vi "Access Integer.vi"(7 "Get/Set":enum16{"Get", "Set"}(ring), 8 "error in (no error)":errorcluster, 9 "Value in":i32, 10 "Key":string, 11 "FlexWorktable in":refnum<class "FlexWorktable.lvclass">) -> (0 "error out":errorcluster, 1 "Value out":i32, 3 "FlexWorktable out":refnum<class "FlexWorktable.lvclass">)   [LabVIEW 2017, in "FlexWorktable.lvclass"]
uses:
  FlexWorktable.lvclass
  FlexWorktable.lvclass/FlexWorktable.ctl
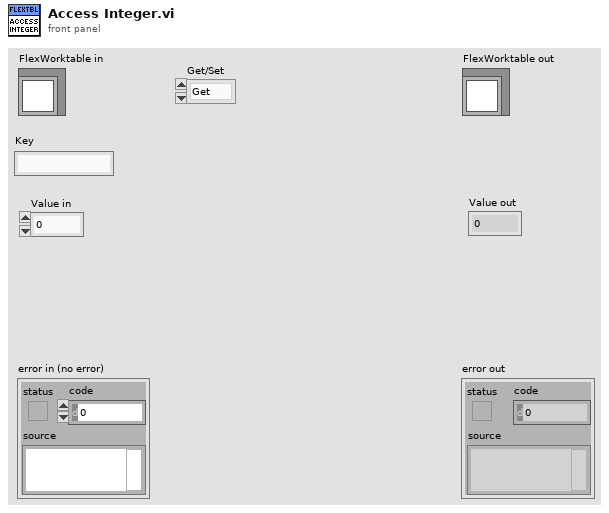
[diagram p1: front panel]
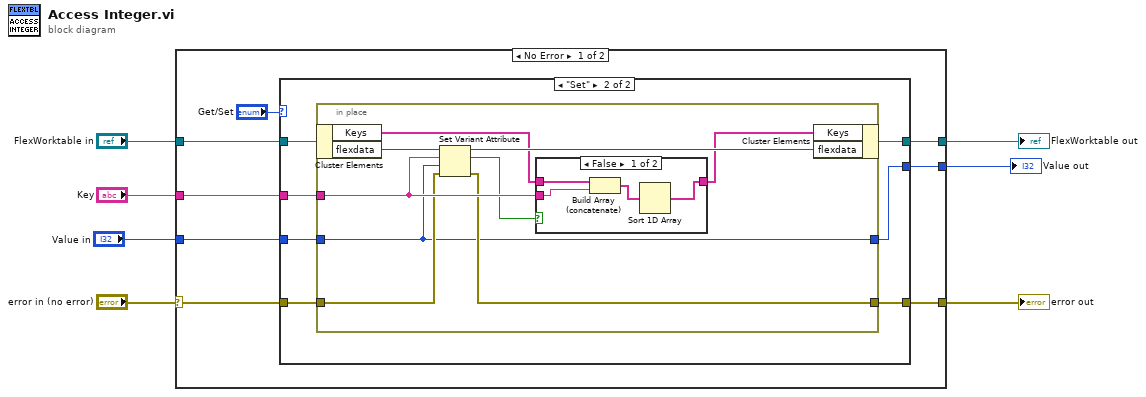
[diagram p0: block diagram]
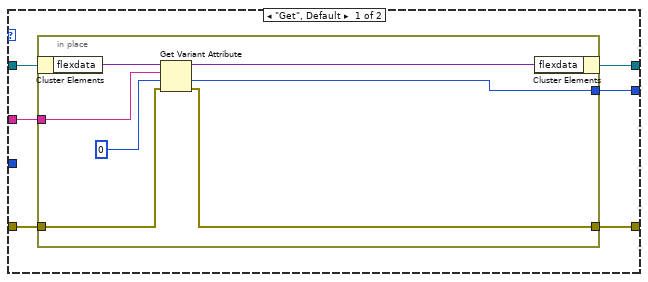
[diagram p2: hidden frame]
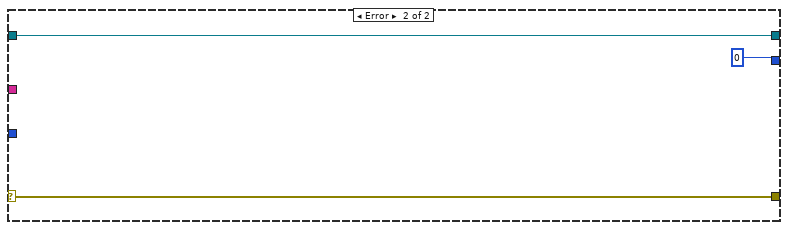
[diagram p4: hidden frame]
diagram:
  n1 = case shown="No Error" "error in (no error)" {
    selector: "error in (no error)" -> [w14 w52]
    tunnel: [w11 w52] -> w4
    tunnel: [w10 w51] -> w6
    tunnel: "FlexWorktable in" -> [w15 w51]
    tunnel: "Key" -> [w13 _]
    tunnel: "Value in" -> [w12 _]
    tunnel: [w8 0] -> w1
    frame No Error {
      n2 = case shown="\"Set\"" "Get/Set" {
        tunnel: w15 -> [w21 w35]
        tunnel: w14 -> [w19 w34]
        tunnel: w13 -> [w20 w33]
        tunnel: w12 -> [_ w32]
        tunnel: [w17 w31] -> w11
        tunnel: [w18 w30] -> w10
        tunnel: [w16 w29] -> w8
        frame "Get", Default {
          n3 = in-place {
            in-place-border: w19 -> [w24]
            in-place-border: w20 -> [w27]
            in-place-border: [w25] -> w17
            in-place-border: [w23] -> w16
            n4 = in-place-cluster #1(w21) -> ("flexdata"=w28:variant)
            n5 = Get Variant Attribute(Variant=w28, name=w27, default value (empty Variant)=0, error in=w24) -> (duplicate Variant=w26:variant, value=w23:i32, error out=w25:errorcluster)  [unwired: 1 out]
            n6 = in-place-cluster #1("flexdata"=w26) -> (w18:refnum<class "FlexWorktable.lvclass">)
          }
        }
        frame "Set" {
          n7 = in-place {
            in-place-border: w34 -> [w40]
            in-place-border: w33 -> [w41]
            in-place-border: w32 -> [w36]
            in-place-border: [w39] -> w31
            in-place-border: [w36] -> w29
            n8 = in-place-cluster #2(w35) -> ("Keys"=w42:string[], "flexdata"=w44:variant)
            n9 = Set Variant Attribute(Variant=w44, name=w41, value=w36, error in=w40) -> (Variant out=w43:variant, replaced=w38:bool, error out=w39:errorcluster)
            n10 = case shown="False" w38 {
              tunnel: w42 -> [w48 w49]
              tunnel: w41 -> [w47 _]
              tunnel: [w45 w49] -> w37
              frame False {
                n11 = Build Array (concatenate)(w48, w47) -> (w46:string[])
                n12 = Sort 1D Array(array=w46) -> (sorted array=w45:string[])
              }
              frame True {
              }
            }
            n13 = in-place-cluster #2("Keys"=w37, "flexdata"=w43) -> (w30:refnum<class "FlexWorktable.lvclass">)
          }
        }
      }
    }
    frame Error {
    }
  }
  "error out" <- w4
  "FlexWorktable out" <- w6
  "Value out" <- w1
